vi "ActionVIOnDownload - Set Scan Rate.vi"(5 "System Definition Dir":path, 6 "IP address":string, 7 "Details Ref":refnum<vi>, 8 "error in (no error)":errorcluster, 10 "WebDAV session in":T1, 11 "Device Item Ref in":T2 format="%.0x") -> (0 "error out":errorcluster, 2 "WebDAV session out":T1, 3 "Device Item Ref out":T2 format="%.0x")   [LabVIEW 2024, in "SEECD System Explorer.lvlib"]
uses:
  SEECD System Explorer.lvlib
  <vilib>/NI VeriStand/Custom Device API/Custom Device Item Ref.ctl
  <vilib>/WebDAVClient/Advanced/SessionHandle.ctl
  <vilib>/NI VeriStand/Custom Device API/Custom Device API.lvlib
  <vilib>/WebDAVClient/NI_WebDAV.lvlib
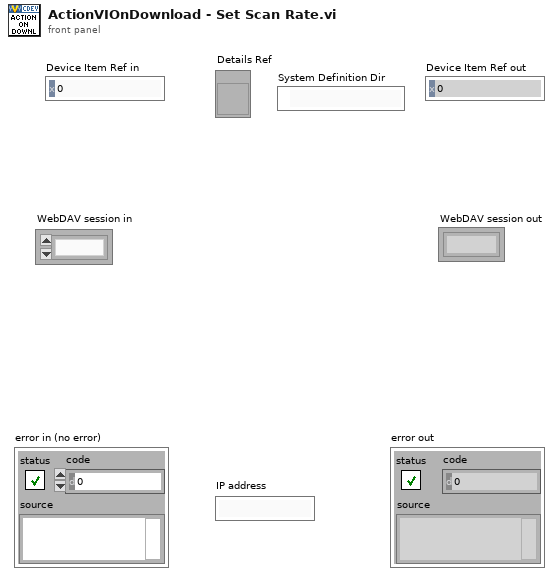
[diagram p1: front panel]
types:
  T1 = typedef "NI_WebDAV.lvlib/SessionHandle.ctl" = refnum<k1>
  T2 = typedef "Custom Device API.lvlib/Custom Device Item Ref.ctl" = u64
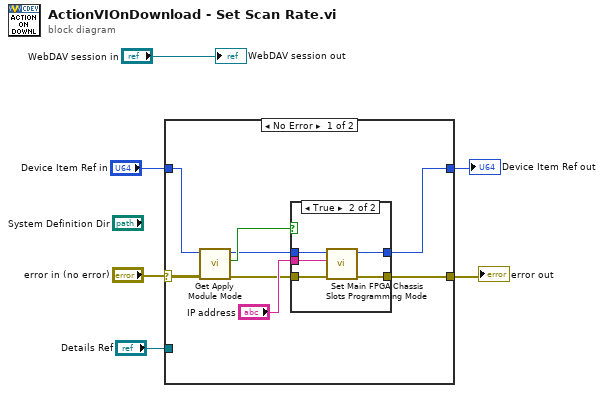
[diagram p0: block diagram]
diagram:
  n1 = case shown="No Error" "error in (no error)" {
    selector: "error in (no error)" -> [w13 w23]
    tunnel: [w8 w23] -> w1
    tunnel: "Device Item Ref in" -> [w12 w22]
    tunnel: [w7 w22] -> w2
    tunnel: "Details Ref" -> [_ _]
    frame No Error {
      n2 = call "Get Apply Module Mode.vi"("error in (no error)"=w13, "Device Item Ref in"=w12) -> ("error out"=w11:errorcluster, "Apply Module Mode"=w10:bool, "Device Item Ref out"=w9:T2)  [unwired: 7 in]
      n3 = case shown="True" w10 {
        tunnel: w9 -> [w16 w21]
        tunnel: "IP address" -> [_ w20]
        tunnel: [w15 w19] -> w8
        tunnel: [w16 w18] -> w7
        tunnel: w11 -> [w15 w17]
        frame False {
        }
        frame True {
          n4 = call "Set Main FPGA Chassis Slots Programming Mode.vi"("error in (no error)"=w17, "serverName in"=w20, "Item Ref in"=w21) -> ("error out"=w19:errorcluster, "Item Ref out"=w18:T2)  [unwired: 6 in, 1 out]
        }
      }
    }
    frame Error {
    }
  }
  "error out" <- w1
  "Device Item Ref out" <- w2
  "WebDAV session out" <- "WebDAV session in"
